vi "Parameter Set.vi"(0 "Device Type":string, 1 "Model Name":string, 3 "Interface":string(combo), 4 "Index Num":string, 5 "Parameter":string, 6 "Interface":string, 7 "Model":string) -> (2 "Data out":string[](array[string]))   [LabVIEW 2018]
panel:
  in  "Cancel":bool
  in  "OK":bool
  out "布尔 2":bool
  out "布尔":bool
  in  "Bar":bool
  in  "Address":string(combo)="1"
  in  "IP":string
  in  "IP 4":string
  in  "IP 3":string
  in  "IP 2":string
  in  "IP":string
  in  "Device Num":string(combo)="1"
  in  "Boolean":bool
  in  "Index Num":string(combo)="1"
  in  "SN":string
  in  "PID":string
  in  "VID":string
  in  "Stop Bits":string(combo)="1"
  in  "Data Bits":string(combo)="8"
  in  "Parity":u16(ring) items=["None", "Odd", "Even", "Mark", "Space"]
  in  "Baud Rate":string(combo)="9600"
  in  "COM Port":string(combo)="1"
  in  "GPIB Address":u16
  # "Drive_Parameter set"
  # "Parameter"
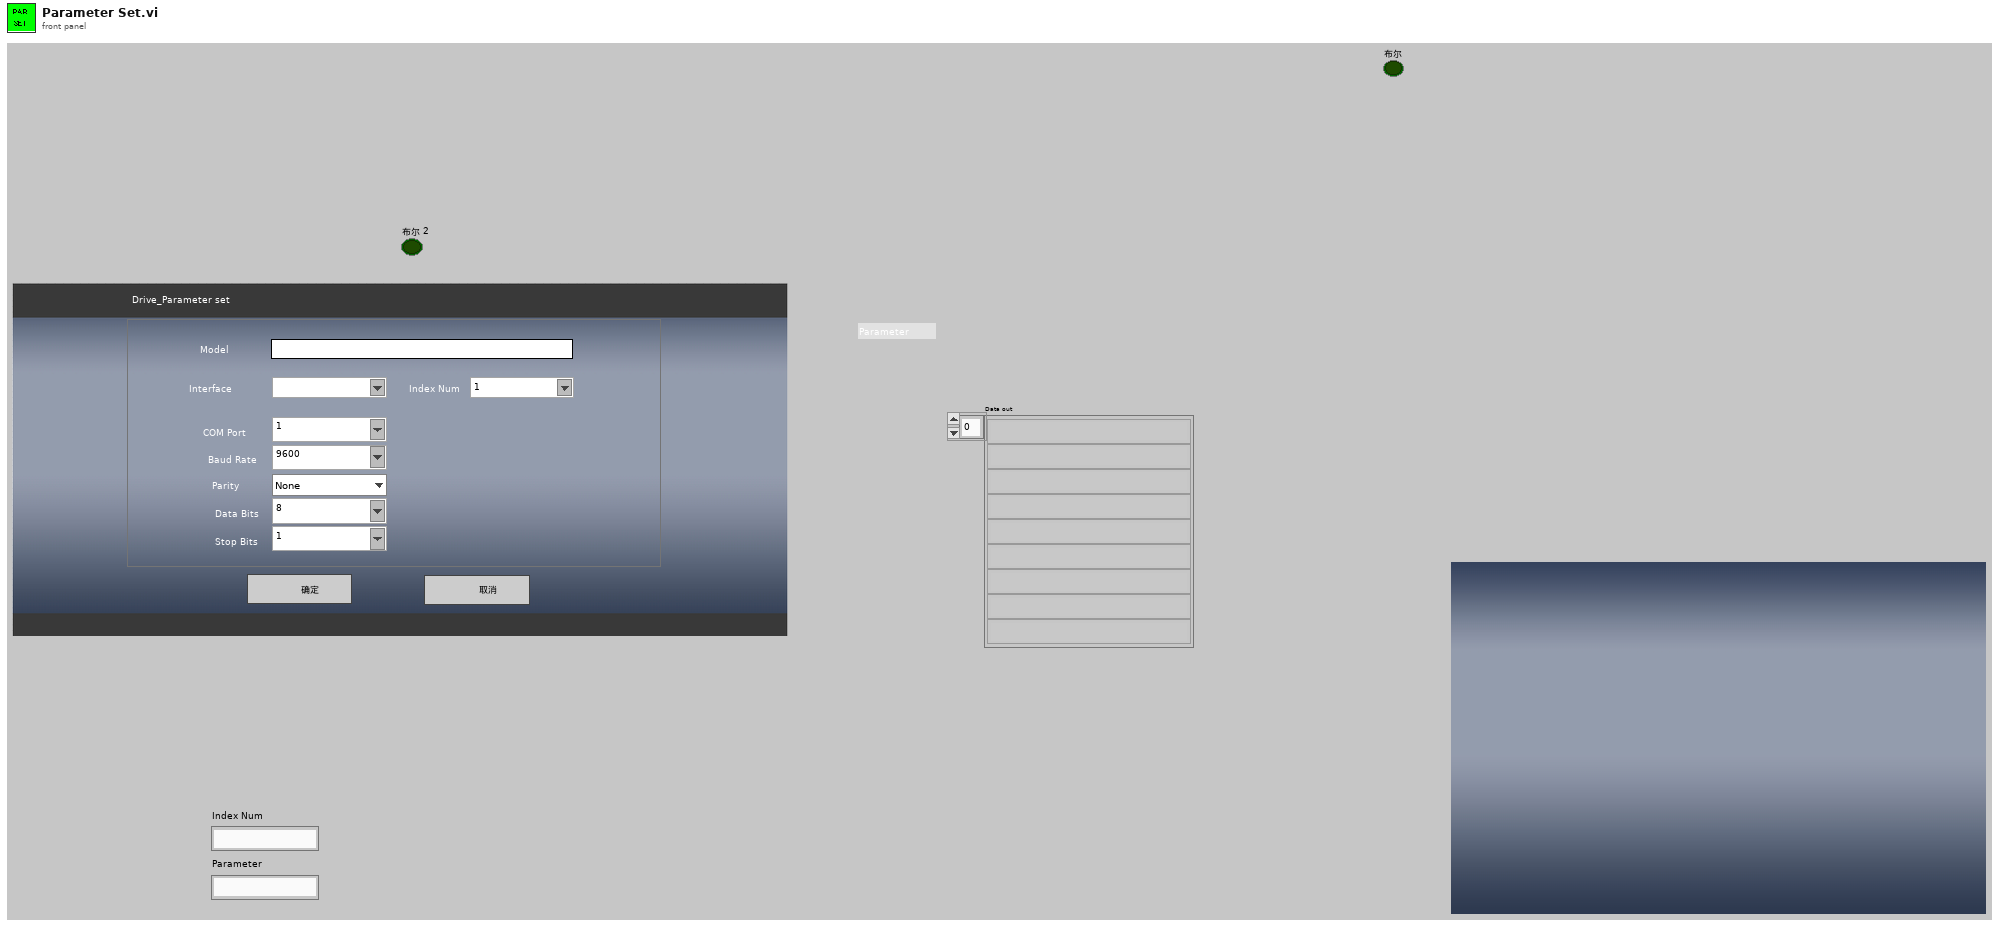
[diagram p1: front panel]
types:
  T1 = typedef "Window Refnum.ctl" = refnum<k1>
  T2 = typedef "Window Rectangle.ctl" = cluster{"left":i16, "top":i16, "right":i16, "bottom":i16}
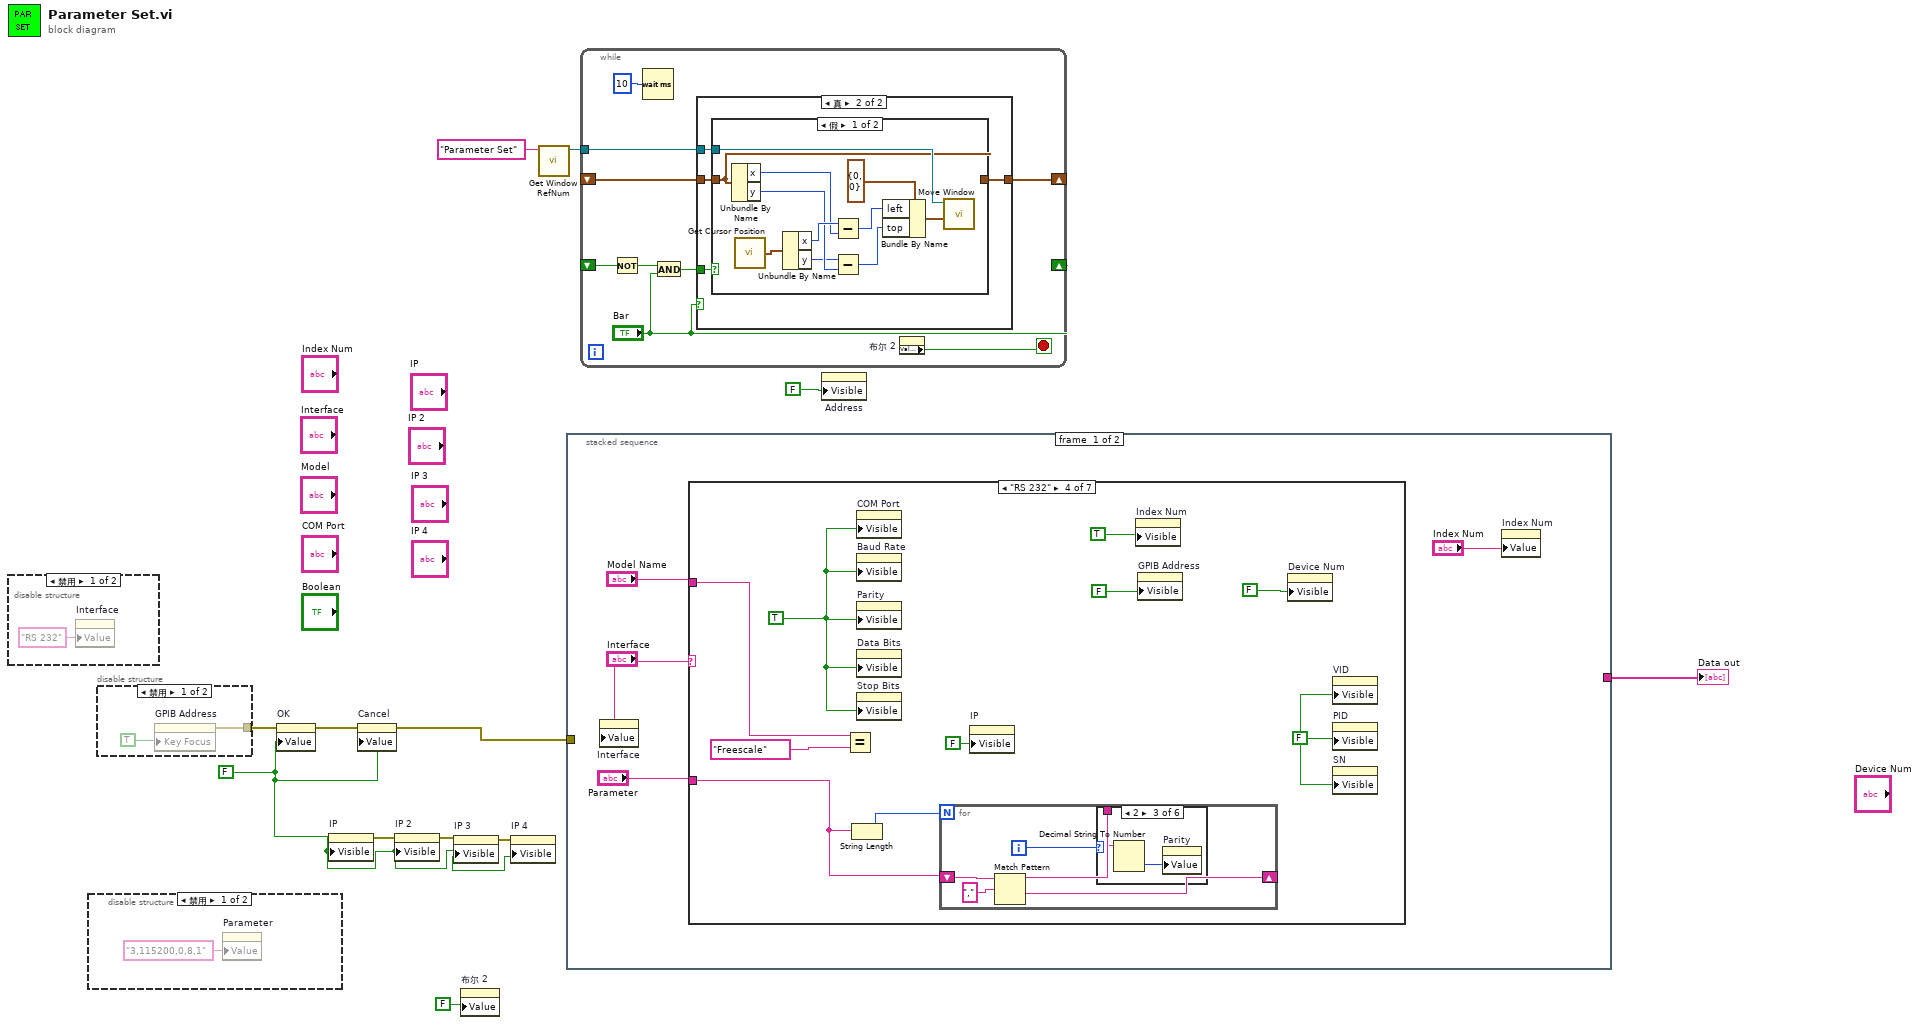
[diagram p0: block diagram]
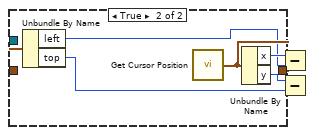
[diagram p6: hidden frame]
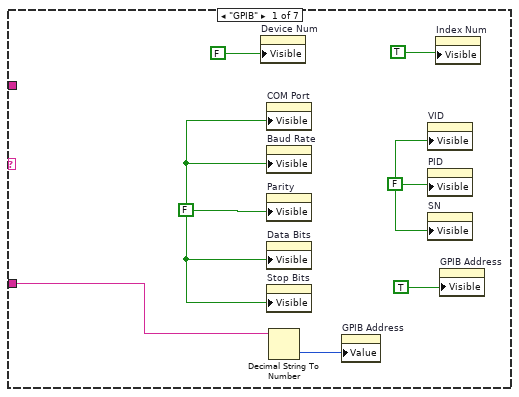
[diagram p7: hidden frame]
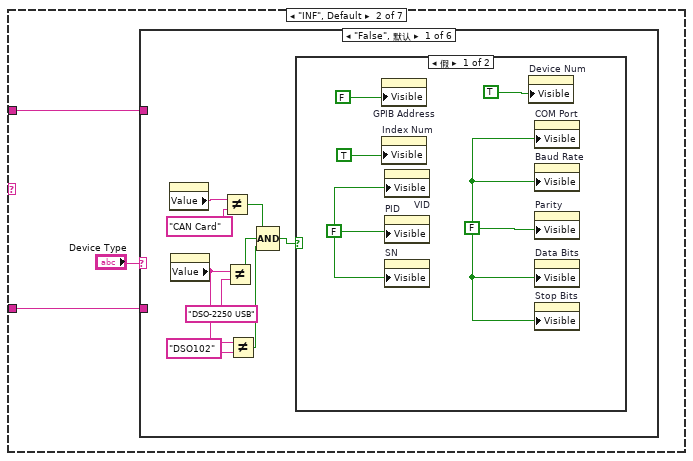
[diagram p8: hidden frame]
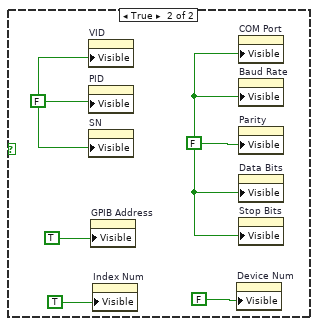
[diagram p9: hidden frame]
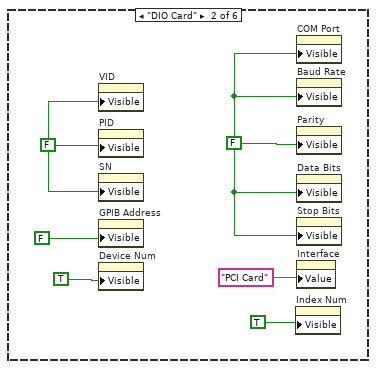
[diagram p10: hidden frame]
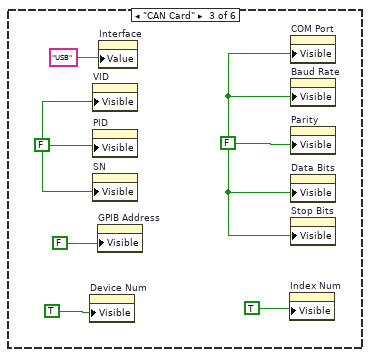
[diagram p11: hidden frame]
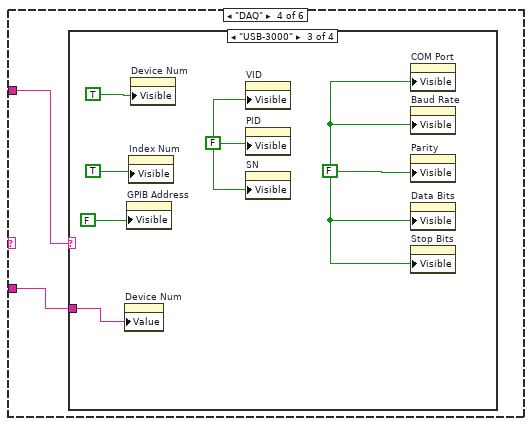
[diagram p12: hidden frame]
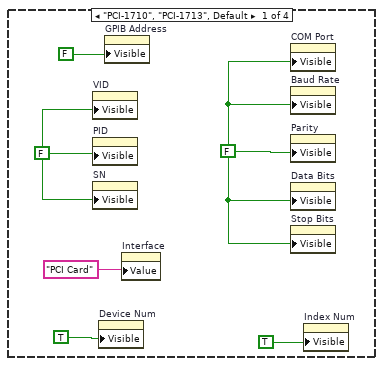
[diagram p13: hidden frame]
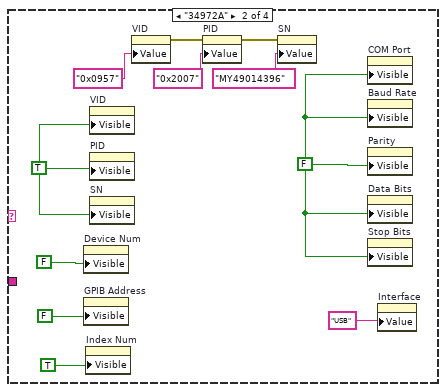
[diagram p14: hidden frame]
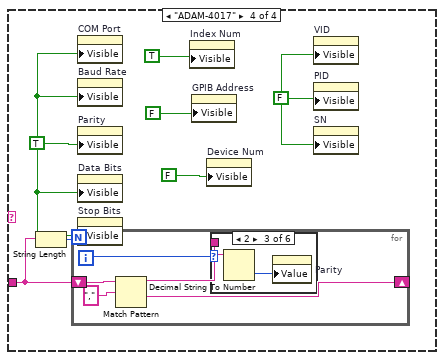
[diagram p15: hidden frame]
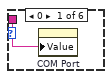
[diagram p16: hidden frame]
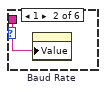
[diagram p17: hidden frame]
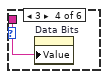
[diagram p18: hidden frame]
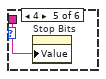
[diagram p19: hidden frame]
diagram:
  w5 = FALSE
  n1 = disable-structure shown="禁用" {
    frame Disabled {
      n2 = property on="Interface" class="Str"("Value"="RS 232" ("Interface")) -> ()  [unwired: 2 in, 2 out]
    }
    frame Enabled {
    }
  }
  n3 = disable-structure shown="禁用" {
    frame Disabled {
      n4 = property on="Parameter" class="Str"("Value"="3,115200,0,8,1" ("Parameter")) -> ()  [unwired: 2 in, 2 out]
    }
    frame Enabled {
    }
  }
  n5 = disable-structure shown="禁用" {
    disable-tunnel: [w16 _] -> w11
    frame Disabled {
      n6 = property on="GPIB Address" class="DigNum (严格)"("Key Focus"=TRUE) -> (error out=w16:errorcluster)  [unwired: 2 in, 1 out]
    }
    frame Enabled {
    }
  }
  n7 = property on="OK" class="Bool (严格)"(error in=w11, "Value"=w5) -> (error out=w12:errorcluster)  [unwired: 1 in, 1 out]
  n8 = property on="IP" class="Str"("Visible"=w5) -> (error out=w6:errorcluster)  [unwired: 2 in, 1 out]
  n9 = property on="Cancel" class="Bool (严格)"(error in=w12, "Value"=w5) -> (error out=w10:errorcluster)  [unwired: 1 in, 1 out]
  n10 = property on="IP 2" class="Str"(error in=w6, "Visible"=w5) -> (error out=w7:errorcluster)  [unwired: 1 in, 1 out]
  n11 = property on="IP 3" class="Str"(error in=w7, "Visible"=w5) -> (error out=w8:errorcluster)  [unwired: 1 in, 1 out]
  n12 = property on="布尔 2" class="Bool (严格)"("Value"=FALSE ("布尔 2")) -> ()  [unwired: 2 in, 2 out]
  n13 = property on="IP 4" class="Str"(error in=w8, "Visible"=w5) -> ()  [unwired: 1 in, 2 out]
  n14 = call "Get Window RefNum.vi"("window name (\"\")"="Parameter Set" ("window name (\"\")")) -> ("window refnum (NaWR)"=w2:T1)  [unwired: 1 in, 7 out]
  n15 = stacked-sequence {
    tunnel: w10 -> [_ w226]
    tunnel: [_ w225] -> w9
    frame #0 {
      n16 = property on="Interface" class="CmbBox"("Value"="Interface") -> ()  [unwired: 2 in, 2 out]
      n17 = case shown="\"RS 232\"" "Interface" {
        tunnel: "Parameter" -> [w23 w28 _ w149 w171 w198 w224]
        tunnel: "Model Name" -> [_ w29 _ w146 w168 w187 _]
        frame "GPIB" {
          w27 = FALSE
          w25 = FALSE
          n18 = property on="Device Num" class="CmbBox"("Visible"=FALSE) -> ()  [unwired: 2 in, 2 out]
          n19 = property on="COM Port" class="CmbBox"("Visible"=w25) -> ()  [unwired: 2 in, 2 out]
          n20 = property on="Baud Rate" class="CmbBox"("Visible"=w25) -> ()  [unwired: 2 in, 2 out]
          n21 = property on="Parity" class="Ring (严格)"("Visible"=w25) -> ()  [unwired: 2 in, 2 out]
          n22 = property on="Data Bits" class="CmbBox"("Visible"=w25) -> ()  [unwired: 2 in, 2 out]
          n23 = property on="Stop Bits" class="CmbBox"("Visible"=w25) -> ()  [unwired: 2 in, 2 out]
          n24 = Decimal String To Number(string=w23) -> (number=w24:i32)  [unwired: 3 out]
          n25 = property on="GPIB Address" class="DigNum (严格)"("Value"=w24) -> ()  [unwired: 2 in, 2 out]
          n26 = property on="VID" class="Str"("Visible"=w27) -> ()  [unwired: 2 in, 2 out]
          n27 = property on="PID" class="Str"("Visible"=w27) -> ()  [unwired: 2 in, 2 out]
          n28 = property on="SN" class="Str"("Visible"=w27) -> ()  [unwired: 2 in, 2 out]
          n29 = property on="Index Num" class="CmbBox"("Visible"=TRUE) -> ()  [unwired: 2 in, 2 out]
          n30 = property on="GPIB Address" class="DigNum (严格)"("Visible"=TRUE) -> ()  [unwired: 2 in, 2 out]
        }
        frame "INF", Default {
          n31 = case shown="\"False\", 默认" "Device Type" {
            tunnel: w29 -> [_ _ _ w63 w105 w117]
            tunnel: w28 -> [_ _ _ w62 _ _]
            frame "False", Default {
              n32 = property on="Device Type" class="Str"() -> ("Value"=w37:string)  [unwired: 2 in, 2 out]
              n33 = property on="Model Name" class="Str"() -> ("Value"=w34:string)  [unwired: 2 in, 2 out]
              n34 = Not Equal?(x=w37, y="CAN Card") -> (x != y?=w36:bool)
              n35 = Not Equal?(x=w34, y="DSO-2250 USB") -> (x != y?=w35:bool)
              n36 = Not Equal?(x=w34, y="DSO102") -> (x != y?=w32:bool)
              n37 = Compound Arithmetic op=AND(w36, w35, w32) -> (w31:bool)
              n38 = case shown="假" w31 {
                frame False {
                  w43 = FALSE
                  w44 = FALSE
                  n39 = property on="GPIB Address" class="DigNum (严格)"("Visible"=FALSE) -> ()  [unwired: 2 in, 2 out]
                  n40 = property on="Index Num" class="CmbBox"("Visible"=TRUE) -> ()  [unwired: 2 in, 2 out]
                  n41 = property on="VID" class="Str"("Visible"=w44) -> ()  [unwired: 2 in, 2 out]
                  n42 = property on="PID" class="Str"("Visible"=w44) -> ()  [unwired: 2 in, 2 out]
                  n43 = property on="SN" class="Str"("Visible"=w44) -> ()  [unwired: 2 in, 2 out]
                  n44 = property on="Device Num" class="CmbBox"("Visible"=TRUE) -> ()  [unwired: 2 in, 2 out]
                  n45 = property on="COM Port" class="CmbBox"("Visible"=w43) -> ()  [unwired: 2 in, 2 out]
                  n46 = property on="Baud Rate" class="CmbBox"("Visible"=w43) -> ()  [unwired: 2 in, 2 out]
                  n47 = property on="Parity" class="Ring (严格)"("Visible"=w43) -> ()  [unwired: 2 in, 2 out]
                  n48 = property on="Data Bits" class="CmbBox"("Visible"=w43) -> ()  [unwired: 2 in, 2 out]
                  n49 = property on="Stop Bits" class="CmbBox"("Visible"=w43) -> ()  [unwired: 2 in, 2 out]
                }
                frame True {
                  w48 = FALSE
                  w49 = FALSE
                  n50 = property on="VID" class="Str"("Visible"=w49) -> ()  [unwired: 2 in, 2 out]
                  n51 = property on="PID" class="Str"("Visible"=w49) -> ()  [unwired: 2 in, 2 out]
                  n52 = property on="SN" class="Str"("Visible"=w49) -> ()  [unwired: 2 in, 2 out]
                  n53 = property on="GPIB Address" class="DigNum (严格)"("Visible"=TRUE) -> ()  [unwired: 2 in, 2 out]
                  n54 = property on="Index Num" class="CmbBox"("Visible"=TRUE) -> ()  [unwired: 2 in, 2 out]
                  n55 = property on="Device Num" class="CmbBox"("Visible"=FALSE) -> ()  [unwired: 2 in, 2 out]
                  n56 = property on="COM Port" class="CmbBox"("Visible"=w48) -> ()  [unwired: 2 in, 2 out]
                  n57 = property on="Baud Rate" class="CmbBox"("Visible"=w48) -> ()  [unwired: 2 in, 2 out]
                  n58 = property on="Parity" class="Ring (严格)"("Visible"=w48) -> ()  [unwired: 2 in, 2 out]
                  n59 = property on="Data Bits" class="CmbBox"("Visible"=w48) -> ()  [unwired: 2 in, 2 out]
                  n60 = property on="Stop Bits" class="CmbBox"("Visible"=w48) -> ()  [unwired: 2 in, 2 out]
                }
              }
            }
            frame "DIO Card" {
              w54 = FALSE
              w55 = FALSE
              n61 = property on="VID" class="Str"("Visible"=w55) -> ()  [unwired: 2 in, 2 out]
              n62 = property on="PID" class="Str"("Visible"=w55) -> ()  [unwired: 2 in, 2 out]
              n63 = property on="SN" class="Str"("Visible"=w55) -> ()  [unwired: 2 in, 2 out]
              n64 = property on="GPIB Address" class="DigNum (严格)"("Visible"=FALSE) -> ()  [unwired: 2 in, 2 out]
              n65 = property on="Device Num" class="CmbBox"("Visible"=TRUE) -> ()  [unwired: 2 in, 2 out]
              n66 = property on="Index Num" class="CmbBox"("Visible"=TRUE) -> ()  [unwired: 2 in, 2 out]
              n67 = property on="COM Port" class="CmbBox"("Visible"=w54) -> ()  [unwired: 2 in, 2 out]
              n68 = property on="Baud Rate" class="CmbBox"("Visible"=w54) -> ()  [unwired: 2 in, 2 out]
              n69 = property on="Parity" class="Ring (严格)"("Visible"=w54) -> ()  [unwired: 2 in, 2 out]
              n70 = property on="Data Bits" class="CmbBox"("Visible"=w54) -> ()  [unwired: 2 in, 2 out]
              n71 = property on="Stop Bits" class="CmbBox"("Visible"=w54) -> ()  [unwired: 2 in, 2 out]
              n72 = property on="Interface" class="CmbBox"("Value"="PCI Card" ("Interface")) -> ()  [unwired: 2 in, 2 out]
            }
            frame "CAN Card" {
              w60 = FALSE
              w61 = FALSE
              n73 = property on="Device Num" class="CmbBox"("Visible"=TRUE) -> ()  [unwired: 2 in, 2 out]
              n74 = property on="VID" class="Str"("Visible"=w61) -> ()  [unwired: 2 in, 2 out]
              n75 = property on="PID" class="Str"("Visible"=w61) -> ()  [unwired: 2 in, 2 out]
              n76 = property on="SN" class="Str"("Visible"=w61) -> ()  [unwired: 2 in, 2 out]
              n77 = property on="GPIB Address" class="DigNum (严格)"("Visible"=FALSE) -> ()  [unwired: 2 in, 2 out]
              n78 = property on="Interface" class="CmbBox"("Value"="USB" ("Interface")) -> ()  [unwired: 2 in, 2 out]
              n79 = property on="Index Num" class="CmbBox"("Visible"=TRUE) -> ()  [unwired: 2 in, 2 out]
              n80 = property on="COM Port" class="CmbBox"("Visible"=w60) -> ()  [unwired: 2 in, 2 out]
              n81 = property on="Baud Rate" class="CmbBox"("Visible"=w60) -> ()  [unwired: 2 in, 2 out]
              n82 = property on="Parity" class="Ring (严格)"("Visible"=w60) -> ()  [unwired: 2 in, 2 out]
              n83 = property on="Data Bits" class="CmbBox"("Visible"=w60) -> ()  [unwired: 2 in, 2 out]
              n84 = property on="Stop Bits" class="CmbBox"("Visible"=w60) -> ()  [unwired: 2 in, 2 out]
            }
            frame "DAQ" {
              n85 = case shown="\"USB-3000\"" w63 {
                tunnel: w62 -> [_ _ w81 w87]
                frame "PCI-1710", "PCI-1713", Default {
                  w68 = FALSE
                  w69 = FALSE
                  n86 = property on="VID" class="Str"("Visible"=w69) -> ()  [unwired: 2 in, 2 out]
                  n87 = property on="PID" class="Str"("Visible"=w69) -> ()  [unwired: 2 in, 2 out]
                  n88 = property on="SN" class="Str"("Visible"=w69) -> ()  [unwired: 2 in, 2 out]
                  n89 = property on="Device Num" class="CmbBox"("Visible"=TRUE) -> ()  [unwired: 2 in, 2 out]
                  n90 = property on="GPIB Address" class="DigNum (严格)"("Visible"=FALSE) -> ()  [unwired: 2 in, 2 out]
                  n91 = property on="Interface" class="CmbBox"("Value"="PCI Card" ("Interface")) -> ()  [unwired: 2 in, 2 out]
                  n92 = property on="COM Port" class="CmbBox"("Visible"=w68) -> ()  [unwired: 2 in, 2 out]
                  n93 = property on="Baud Rate" class="CmbBox"("Visible"=w68) -> ()  [unwired: 2 in, 2 out]
                  n94 = property on="Parity" class="Ring (严格)"("Visible"=w68) -> ()  [unwired: 2 in, 2 out]
                  n95 = property on="Data Bits" class="CmbBox"("Visible"=w68) -> ()  [unwired: 2 in, 2 out]
                  n96 = property on="Stop Bits" class="CmbBox"("Visible"=w68) -> ()  [unwired: 2 in, 2 out]
                  n97 = property on="Index Num" class="CmbBox"("Visible"=TRUE) -> ()  [unwired: 2 in, 2 out]
                }
                frame "34972A" {
                  w79 = FALSE
                  w80 = TRUE
                  n98 = property on="Device Num" class="CmbBox"("Visible"=FALSE) -> ()  [unwired: 2 in, 2 out]
                  n99 = property on="GPIB Address" class="DigNum (严格)"("Visible"=FALSE) -> ()  [unwired: 2 in, 2 out]
                  n100 = property on="Index Num" class="CmbBox"("Visible"=TRUE) -> ()  [unwired: 2 in, 2 out]
                  n101 = property on="VID" class="Str"("Visible"=w80) -> ()  [unwired: 2 in, 2 out]
                  n102 = property on="PID" class="Str"("Visible"=w80) -> ()  [unwired: 2 in, 2 out]
                  n103 = property on="SN" class="Str"("Visible"=w80) -> ()  [unwired: 2 in, 2 out]
                  n104 = property on="VID" class="Str"("Value"="0x0957" ("VID")) -> (error out=w75:errorcluster)  [unwired: 2 in, 1 out]
                  n105 = property on="PID" class="Str"(error in=w75, "Value"="0x2007" ("PID")) -> (error out=w73:errorcluster)  [unwired: 1 in, 1 out]
                  n106 = property on="SN" class="Str"(error in=w73, "Value"="MY49014396" ("SN")) -> ()  [unwired: 1 in, 2 out]
                  n107 = property on="COM Port" class="CmbBox"("Visible"=w79) -> ()  [unwired: 2 in, 2 out]
                  n108 = property on="Baud Rate" class="CmbBox"("Visible"=w79) -> ()  [unwired: 2 in, 2 out]
                  n109 = property on="Parity" class="Ring (严格)"("Visible"=w79) -> ()  [unwired: 2 in, 2 out]
                  n110 = property on="Data Bits" class="CmbBox"("Visible"=w79) -> ()  [unwired: 2 in, 2 out]
                  n111 = property on="Stop Bits" class="CmbBox"("Visible"=w79) -> ()  [unwired: 2 in, 2 out]
                  n112 = property on="Interface" class="CmbBox"("Value"="USB" ("Interface")) -> ()  [unwired: 2 in, 2 out]
                }
                frame "USB-3000" {
                  w83 = FALSE
                  w84 = FALSE
                  n113 = property on="Device Num" class="CmbBox"("Value"=w81) -> ()  [unwired: 2 in, 2 out]
                  n114 = property on="GPIB Address" class="DigNum (严格)"("Visible"=FALSE) -> ()  [unwired: 2 in, 2 out]
                  n115 = property on="Index Num" class="CmbBox"("Visible"=TRUE) -> ()  [unwired: 2 in, 2 out]
                  n116 = property on="Device Num" class="CmbBox"("Visible"=TRUE) -> ()  [unwired: 2 in, 2 out]
                  n117 = property on="VID" class="Str"("Visible"=w83) -> ()  [unwired: 2 in, 2 out]
                  n118 = property on="PID" class="Str"("Visible"=w83) -> ()  [unwired: 2 in, 2 out]
                  n119 = property on="SN" class="Str"("Visible"=w83) -> ()  [unwired: 2 in, 2 out]
                  n120 = property on="COM Port" class="CmbBox"("Visible"=w84) -> ()  [unwired: 2 in, 2 out]
                  n121 = property on="Baud Rate" class="CmbBox"("Visible"=w84) -> ()  [unwired: 2 in, 2 out]
                  n122 = property on="Parity" class="Ring (严格)"("Visible"=w84) -> ()  [unwired: 2 in, 2 out]
                  n123 = property on="Data Bits" class="CmbBox"("Visible"=w84) -> ()  [unwired: 2 in, 2 out]
                  n124 = property on="Stop Bits" class="CmbBox"("Visible"=w84) -> ()  [unwired: 2 in, 2 out]
                }
                frame "ADAM-4017" {
                  w91 = FALSE
                  w93 = TRUE
                  n125 = String Length(string=w87) -> (length=w88:i32)
                  n126 = for {
                    N: w88 -> [_]
                    shift-right: [w96] -> _
                    shift-left: w87 -> [w98]
                    i -> [w95]
                    n127 = Match Pattern(string=w98, regular expression=",") -> (before substring=w94:string, after substring=w96:string)  [unwired: 3 out]
                    n128 = case shown="2" w95 {
                      tunnel: w94 -> [w99 w100 w102 w103 w104 _]
                      frame 0 {
                        n129 = property on="COM Port" class="CmbBox"("Value"=w99) -> ()  [unwired: 2 in, 2 out]
                      }
                      frame 1 {
                        n130 = property on="Baud Rate" class="CmbBox"("Value"=w100) -> ()  [unwired: 2 in, 2 out]
                      }
                      frame 2 {
                        n131 = Decimal String To Number(string=w102) -> (number=w101:i32)  [unwired: 3 out]
                        n132 = property on="Parity" class="Ring (严格)"("Value"=w101) -> ()  [unwired: 2 in, 2 out]
                      }
                      frame 3 {
                        n133 = property on="Data Bits" class="CmbBox"("Value"=w103) -> ()  [unwired: 2 in, 2 out]
                      }
                      frame 4 {
                        n134 = property on="Stop Bits" class="CmbBox"("Value"=w104) -> ()  [unwired: 2 in, 2 out]
                      }
                      frame 5, Default {
                      }
                    }
                  }
                  n135 = property on="COM Port" class="CmbBox"("Visible"=w93) -> ()  [unwired: 2 in, 2 out]
                  n136 = property on="Baud Rate" class="CmbBox"("Visible"=w93) -> ()  [unwired: 2 in, 2 out]
                  n137 = property on="Parity" class="Ring (严格)"("Visible"=w93) -> ()  [unwired: 2 in, 2 out]
                  n138 = property on="Data Bits" class="CmbBox"("Visible"=w93) -> ()  [unwired: 2 in, 2 out]
                  n139 = property on="Stop Bits" class="CmbBox"("Visible"=w93) -> ()  [unwired: 2 in, 2 out]
                  n140 = property on="Index Num" class="CmbBox"("Visible"=TRUE) -> ()  [unwired: 2 in, 2 out]
                  n141 = property on="GPIB Address" class="DigNum (严格)"("Visible"=FALSE) -> ()  [unwired: 2 in, 2 out]
                  n142 = property on="Device Num" class="CmbBox"("Visible"=FALSE) -> ()  [unwired: 2 in, 2 out]
                  n143 = property on="VID" class="Str"("Visible"=w91) -> ()  [unwired: 2 in, 2 out]
                  n144 = property on="PID" class="Str"("Visible"=w91) -> ()  [unwired: 2 in, 2 out]
                  n145 = property on="SN" class="Str"("Visible"=w91) -> ()  [unwired: 2 in, 2 out]
                }
              }
            }
            frame "Power Aanalysis Meter" {
              n146 = case shown="\"66202\"" w105 {
                frame "66202" {
                  w115 = FALSE
                  w116 = TRUE
                  n147 = property on="VID" class="Str"("Visible"=w116) -> ()  [unwired: 2 in, 2 out]
                  n148 = property on="PID" class="Str"("Visible"=w116) -> ()  [unwired: 2 in, 2 out]
                  n149 = property on="SN" class="Str"("Visible"=w116) -> ()  [unwired: 2 in, 2 out]
                  n150 = property on="VID" class="Str"("Value"="0x0A69" ("VID")) -> (error out=w111:errorcluster)  [unwired: 2 in, 1 out]
                  n151 = property on="PID" class="Str"(error in=w111, "Value"="0x0835" ("PID")) -> (error out=w109:errorcluster)  [unwired: 1 in, 1 out]
                  n152 = property on="Device Num" class="CmbBox"("Visible"=FALSE) -> ()  [unwired: 2 in, 2 out]
                  n153 = property on="GPIB Address" class="DigNum (严格)"("Visible"=FALSE) -> ()  [unwired: 2 in, 2 out]
                  n154 = property on="Index Num" class="CmbBox"("Visible"=TRUE) -> ()  [unwired: 2 in, 2 out]
                  n155 = property on="SN" class="Str"(error in=w109, "Value"="A66200110136" ("SN")) -> ()  [unwired: 1 in, 2 out]
                  n156 = property on="COM Port" class="CmbBox"("Visible"=w115) -> ()  [unwired: 2 in, 2 out]
                  n157 = property on="Baud Rate" class="CmbBox"("Visible"=w115) -> ()  [unwired: 2 in, 2 out]
                  n158 = property on="Parity" class="Ring (严格)"("Visible"=w115) -> ()  [unwired: 2 in, 2 out]
                  n159 = property on="Data Bits" class="CmbBox"("Visible"=w115) -> ()  [unwired: 2 in, 2 out]
                  n160 = property on="Stop Bits" class="CmbBox"("Visible"=w115) -> ()  [unwired: 2 in, 2 out]
                  n161 = property on="Interface" class="CmbBox"("Value"="USB" ("Interface")) -> ()  [unwired: 2 in, 2 out]
                }
                frame "false", Default {
                }
              }
            }
            frame "Oscilloscope" {
              n162 = case shown="\"DPO-3054\"" w117 {
                frame "DPO-3054" {
                  w127 = FALSE
                  w128 = TRUE
                  n163 = property on="Device Num" class="CmbBox"("Visible"=FALSE) -> ()  [unwired: 2 in, 2 out]
                  n164 = property on="VID" class="Str"("Visible"=w128) -> ()  [unwired: 2 in, 2 out]
                  n165 = property on="PID" class="Str"("Visible"=w128) -> ()  [unwired: 2 in, 2 out]
                  n166 = property on="SN" class="Str"("Visible"=w128) -> ()  [unwired: 2 in, 2 out]
                  n167 = property on="VID" class="Str"("Value"="0x0699" ("VID")) -> (error out=w123:errorcluster)  [unwired: 2 in, 1 out]
                  n168 = property on="PID" class="Str"(error in=w123, "Value"="0x0415" ("PID")) -> (error out=w121:errorcluster)  [unwired: 1 in, 1 out]
                  n169 = property on="GPIB Address" class="DigNum (严格)"("Visible"=FALSE) -> ()  [unwired: 2 in, 2 out]
                  n170 = property on="Index Num" class="CmbBox"("Visible"=TRUE) -> ()  [unwired: 2 in, 2 out]
                  n171 = property on="SN" class="Str"(error in=w121, "Value"="C030431" ("SN")) -> ()  [unwired: 1 in, 2 out]
                  n172 = property on="COM Port" class="CmbBox"("Visible"=w127) -> ()  [unwired: 2 in, 2 out]
                  n173 = property on="Baud Rate" class="CmbBox"("Visible"=w127) -> ()  [unwired: 2 in, 2 out]
                  n174 = property on="Parity" class="Ring (严格)"("Visible"=w127) -> ()  [unwired: 2 in, 2 out]
                  n175 = property on="Data Bits" class="CmbBox"("Visible"=w127) -> ()  [unwired: 2 in, 2 out]
                  n176 = property on="Stop Bits" class="CmbBox"("Visible"=w127) -> ()  [unwired: 2 in, 2 out]
                  n177 = property on="Interface" class="CmbBox"("Value"="USB" ("Interface")) -> ()  [unwired: 2 in, 2 out]
                }
                frame "TDS 2014C" {
                  w138 = FALSE
                  w139 = TRUE
                  n178 = property on="Interface" class="CmbBox"("Value"="USB" ("Interface")) -> ()  [unwired: 2 in, 2 out]
                  n179 = property on="VID" class="Str"("Visible"=w139) -> ()  [unwired: 2 in, 2 out]
                  n180 = property on="PID" class="Str"("Visible"=w139) -> ()  [unwired: 2 in, 2 out]
                  n181 = property on="SN" class="Str"("Visible"=w139) -> ()  [unwired: 2 in, 2 out]
                  n182 = property on="VID" class="Str"("Value"="0x0699" ("VID")) -> (error out=w134:errorcluster)  [unwired: 2 in, 1 out]
                  n183 = property on="PID" class="Str"(error in=w134, "Value"="0x03A4" ("PID")) -> (error out=w132:errorcluster)  [unwired: 1 in, 1 out]
                  n184 = property on="Device Num" class="CmbBox"("Visible"=FALSE) -> ()  [unwired: 2 in, 2 out]
                  n185 = property on="GPIB Address" class="DigNum (严格)"("Visible"=FALSE) -> ()  [unwired: 2 in, 2 out]
                  n186 = property on="Index Num" class="CmbBox"("Visible"=TRUE) -> ()  [unwired: 2 in, 2 out]
                  n187 = property on="SN" class="Str"(error in=w132, "Value"="C030830" ("SN")) -> ()  [unwired: 1 in, 2 out]
                  n188 = property on="COM Port" class="CmbBox"("Visible"=w138) -> ()  [unwired: 2 in, 2 out]
                  n189 = property on="Baud Rate" class="CmbBox"("Visible"=w138) -> ()  [unwired: 2 in, 2 out]
                  n190 = property on="Parity" class="Ring (严格)"("Visible"=w138) -> ()  [unwired: 2 in, 2 out]
                  n191 = property on="Data Bits" class="CmbBox"("Visible"=w138) -> ()  [unwired: 2 in, 2 out]
                  n192 = property on="Stop Bits" class="CmbBox"("Visible"=w138) -> ()  [unwired: 2 in, 2 out]
                }
                frame "false", Default {
                }
              }
            }
          }
        }
        frame "TCP" {
          w140 = TRUE
          # "读取程式中设定的值到选择框"
          n193 = property on="IP" class="Str"("Visible"=w140) -> (error out=w143:errorcluster)  [unwired: 2 in, 1 out]
          n194 = property on="IP 2" class="Str"(error in=w143, "Visible"=w140) -> (error out=w142:errorcluster)  [unwired: 1 in, 1 out]
          n195 = property on="IP 3" class="Str"(error in=w142, "Visible"=w140) -> (error out=w141:errorcluster)  [unwired: 1 in, 1 out]
          n196 = property on="IP 4" class="Str"(error in=w141, "Visible"=w140) -> ()  [unwired: 1 in, 2 out]
        }
        frame "RS 232" {
          w151 = FALSE
          w153 = TRUE
          n197 = Equal?(x=w146, y="Freescale") -> ()  [unwired: 1 out]
          n198 = String Length(string=w149) -> (length=w150:i32)
          n199 = property on="COM Port" class="CmbBox"("Visible"=w153) -> ()  [unwired: 2 in, 2 out]
          n200 = property on="Baud Rate" class="CmbBox"("Visible"=w153) -> ()  [unwired: 2 in, 2 out]
          n201 = property on="Parity" class="Ring (严格)"("Visible"=w153) -> ()  [unwired: 2 in, 2 out]
          n202 = property on="Data Bits" class="CmbBox"("Visible"=w153) -> ()  [unwired: 2 in, 2 out]
          n203 = property on="Stop Bits" class="CmbBox"("Visible"=w153) -> ()  [unwired: 2 in, 2 out]
          n204 = for {
            N: w150 -> [_]
            shift-right: [w156] -> _
            shift-left: w149 -> [w158]
            i -> [w155]
            n205 = Match Pattern(string=w158, regular expression=",") -> (before substring=w154:string, after substring=w156:string)  [unwired: 3 out]
            n206 = case shown="2" w155 {
              tunnel: w154 -> [w159 w160 w162 w163 w164 _]
              frame 0 {
                n207 = property on="COM Port" class="CmbBox"("Value"=w159) -> ()  [unwired: 2 in, 2 out]
              }
              frame 1 {
                n208 = property on="Baud Rate" class="CmbBox"("Value"=w160) -> ()  [unwired: 2 in, 2 out]
              }
              frame 2 {
                n209 = Decimal String To Number(string=w162) -> (number=w161:i32)  [unwired: 3 out]
                n210 = property on="Parity" class="Ring (严格)"("Value"=w161) -> ()  [unwired: 2 in, 2 out]
              }
              frame 3 {
                n211 = property on="Data Bits" class="CmbBox"("Value"=w163) -> ()  [unwired: 2 in, 2 out]
              }
              frame 4 {
                n212 = property on="Stop Bits" class="CmbBox"("Value"=w164) -> ()  [unwired: 2 in, 2 out]
              }
              frame 5, Default {
              }
            }
          }
          n213 = property on="IP" class="Str"("Visible"=FALSE ("可见")) -> ()  [unwired: 2 in, 2 out]
          n214 = property on="Index Num" class="CmbBox"("Visible"=TRUE) -> ()  [unwired: 2 in, 2 out]
          n215 = property on="GPIB Address" class="DigNum (严格)"("Visible"=FALSE) -> ()  [unwired: 2 in, 2 out]
          n216 = property on="Device Num" class="CmbBox"("Visible"=FALSE) -> ()  [unwired: 2 in, 2 out]
          n217 = property on="VID" class="Str"("Visible"=w151) -> ()  [unwired: 2 in, 2 out]
          n218 = property on="PID" class="Str"("Visible"=w151) -> ()  [unwired: 2 in, 2 out]
          n219 = property on="SN" class="Str"("Visible"=w151) -> ()  [unwired: 2 in, 2 out]
        }
        frame "RS 485" {
          w173 = FALSE
          w165 = TRUE
          n220 = String Length(string=w171) -> (length=w172:i32)
          n221 = Equal?(x=w168, y="Freescale") -> (x = y?=w166:bool)
          n222 = property on="COM Port" class="CmbBox"("Visible"=w165) -> ()  [unwired: 2 in, 2 out]
          n223 = property on="Baud Rate" class="CmbBox"("Visible"=w165) -> ()  [unwired: 2 in, 2 out]
          n224 = property on="Parity" class="Ring (严格)"("Visible"=w165) -> ()  [unwired: 2 in, 2 out]
          n225 = property on="Data Bits" class="CmbBox"("Visible"=w165) -> ()  [unwired: 2 in, 2 out]
          n226 = property on="Stop Bits" class="CmbBox"("Visible"=w165) -> ()  [unwired: 2 in, 2 out]
          n227 = for {
            N: w172 -> [_]
            shift-right: [w177] -> _
            shift-left: w171 -> [w179]
            i -> [w176]
            n228 = Match Pattern(string=w179, regular expression=",") -> (before substring=w175:string, after substring=w177:string)  [unwired: 3 out]
            n229 = case shown="0" w176 {
              tunnel: w175 -> [w180 w181 w183 w184 w185 _]
              frame 0 {
                n230 = property on="COM Port" class="CmbBox"("Value"=w180) -> ()  [unwired: 2 in, 2 out]
              }
              frame 1 {
                n231 = property on="Baud Rate" class="CmbBox"("Value"=w181) -> ()  [unwired: 2 in, 2 out]
              }
              frame 2 {
                n232 = Decimal String To Number(string=w183) -> (number=w182:i32)  [unwired: 3 out]
                n233 = property on="Parity" class="Ring (严格)"("Value"=w182) -> ()  [unwired: 2 in, 2 out]
              }
              frame 3 {
                n234 = property on="Data Bits" class="CmbBox"("Value"=w184) -> ()  [unwired: 2 in, 2 out]
              }
              frame 4 {
                n235 = property on="Stop Bits" class="CmbBox"("Value"=w185) -> ()  [unwired: 2 in, 2 out]
              }
              frame 5, Default {
              }
            }
          }
          n236 = property on="Address" class="CmbBox"("Visible"=w165) -> ()  [unwired: 2 in, 2 out]
          n237 = property on="IP" class="Str"("Visible"=w166) -> ()  [unwired: 2 in, 2 out]
          n238 = property on="Index Num" class="CmbBox"("Visible"=TRUE) -> ()  [unwired: 2 in, 2 out]
          n239 = property on="GPIB Address" class="DigNum (严格)"("Visible"=FALSE) -> ()  [unwired: 2 in, 2 out]
          n240 = property on="Device Num" class="CmbBox"("Visible"=FALSE) -> ()  [unwired: 2 in, 2 out]
          n241 = property on="VID" class="Str"("Visible"=w173) -> ()  [unwired: 2 in, 2 out]
          n242 = property on="PID" class="Str"("Visible"=w173) -> ()  [unwired: 2 in, 2 out]
          n243 = property on="SN" class="Str"("Visible"=w173) -> ()  [unwired: 2 in, 2 out]
        }
        frame "USB" {
          n244 = property on="Device Type" class="Str"() -> ("Value"=w195:string)  [unwired: 2 in, 2 out]
          n245 = property on="Model Name" class="Str"() -> ("Value"=w192:string)  [unwired: 2 in, 2 out]
          n246 = Equal?(x=w187, y="Freescale") -> (x = y?=w186:bool)
          n247 = Not Equal?(x=w195, y="CAN Card") -> (x != y?=w194:bool)
          n248 = Not Equal?(x=w192, y="DSO102") -> (x != y?=w190:bool)
          n249 = Not Equal?(x=w192, y="DSO-2250 USB") -> (x != y?=w193:bool)
          n250 = property on="IP" class="Str"("Visible"=w186) -> ()  [unwired: 2 in, 2 out]
          n251 = Compound Arithmetic op=AND(w194, w193, w190) -> (w189:bool)
          n252 = case shown="真" w189 {
            tunnel: w198 -> [_ w206]
            frame False {
              w201 = FALSE
              w203 = FALSE
              n253 = property on="Index Num" class="CmbBox"("Visible"=TRUE) -> ()  [unwired: 2 in, 2 out]
              n254 = property on="VID" class="Str"("Visible"=w203) -> ()  [unwired: 2 in, 2 out]
              n255 = property on="PID" class="Str"("Visible"=w203) -> ()  [unwired: 2 in, 2 out]
              n256 = property on="SN" class="Str"("Visible"=w203) -> ()  [unwired: 2 in, 2 out]
              n257 = property on="GPIB Address" class="DigNum (严格)"("Visible"=FALSE) -> ()  [unwired: 2 in, 2 out]
              n258 = property on="Device Num" class="CmbBox"("Visible"=TRUE) -> ()  [unwired: 2 in, 2 out]
              n259 = property on="COM Port" class="CmbBox"("Visible"=w201) -> ()  [unwired: 2 in, 2 out]
              n260 = property on="Baud Rate" class="CmbBox"("Visible"=w201) -> ()  [unwired: 2 in, 2 out]
              n261 = property on="Parity" class="Ring (严格)"("Visible"=w201) -> ()  [unwired: 2 in, 2 out]
              n262 = property on="Data Bits" class="CmbBox"("Visible"=w201) -> ()  [unwired: 2 in, 2 out]
              n263 = property on="Stop Bits" class="CmbBox"("Visible"=w201) -> ()  [unwired: 2 in, 2 out]
            }
            frame True {
              w208 = FALSE
              w210 = TRUE
              n264 = String Length(string=w206) -> (length=w207:i32)
              n265 = property on="VID" class="Str"("Visible"=w210) -> ()  [unwired: 2 in, 2 out]
              n266 = property on="PID" class="Str"("Visible"=w210) -> ()  [unwired: 2 in, 2 out]
              n267 = property on="SN" class="Str"("Visible"=w210) -> ()  [unwired: 2 in, 2 out]
              n268 = property on="GPIB Address" class="DigNum (严格)"("Visible"=FALSE) -> ()  [unwired: 2 in, 2 out]
              n269 = for {
                N: w207 -> [_]
                shift-right: [w213] -> _
                shift-left: w206 -> [w215]
                i -> [w212]
                n270 = Match Pattern(string=w215, regular expression=",") -> (before substring=w211:string, after substring=w213:string)  [unwired: 3 out]
                n271 = case shown="0" w212 {
                  tunnel: w211 -> [w216 w217 w218 _ _ _]
                  frame 0 {
                    n272 = property on="VID" class="Str"("Value"=w216) -> ()  [unwired: 2 in, 2 out]
                  }
                  frame 1 {
                    n273 = property on="PID" class="Str"("Value"=w217) -> ()  [unwired: 2 in, 2 out]
                  }
                  frame 2 {
                    n274 = property on="SN" class="Str"("Value"=w218) -> ()  [unwired: 2 in, 2 out]
                  }
                  frame 3 {
                  }
                  frame 4 {
                  }
                  frame 5, Default {
                  }
                }
              }
              n275 = property on="COM Port" class="CmbBox"("Visible"=w208) -> ()  [unwired: 2 in, 2 out]
              n276 = property on="Baud Rate" class="CmbBox"("Visible"=w208) -> ()  [unwired: 2 in, 2 out]
              n277 = property on="Parity" class="Ring (严格)"("Visible"=w208) -> ()  [unwired: 2 in, 2 out]
              n278 = property on="Data Bits" class="CmbBox"("Visible"=w208) -> ()  [unwired: 2 in, 2 out]
              n279 = property on="Stop Bits" class="CmbBox"("Visible"=w208) -> ()  [unwired: 2 in, 2 out]
              n280 = property on="Index Num" class="CmbBox"("Visible"=TRUE) -> ()  [unwired: 2 in, 2 out]
              n281 = property on="Device Num" class="CmbBox"("Visible"=FALSE) -> ()  [unwired: 2 in, 2 out]
            }
          }
        }
        frame "PCI Card" {
          w220 = FALSE
          w221 = FALSE
          n282 = property on="Device Num" class="CmbBox"("Value"=w224) -> ()  [unwired: 2 in, 2 out]
          n283 = property on="GPIB Address" class="DigNum (严格)"("Visible"=FALSE) -> ()  [unwired: 2 in, 2 out]
          n284 = property on="Index Num" class="CmbBox"("Visible"=TRUE) -> ()  [unwired: 2 in, 2 out]
          n285 = property on="Device Num" class="CmbBox"("Visible"=TRUE) -> ()  [unwired: 2 in, 2 out]
          n286 = property on="VID" class="Str"("Visible"=w220) -> ()  [unwired: 2 in, 2 out]
          n287 = property on="PID" class="Str"("Visible"=w220) -> ()  [unwired: 2 in, 2 out]
          n288 = property on="SN" class="Str"("Visible"=w220) -> ()  [unwired: 2 in, 2 out]
          n289 = property on="COM Port" class="CmbBox"("Visible"=w221) -> ()  [unwired: 2 in, 2 out]
          n290 = property on="Baud Rate" class="CmbBox"("Visible"=w221) -> ()  [unwired: 2 in, 2 out]
          n291 = property on="Parity" class="Ring (严格)"("Visible"=w221) -> ()  [unwired: 2 in, 2 out]
          n292 = property on="Data Bits" class="CmbBox"("Visible"=w221) -> ()  [unwired: 2 in, 2 out]
          n293 = property on="Stop Bits" class="CmbBox"("Visible"=w221) -> ()  [unwired: 2 in, 2 out]
        }
      }
      n294 = property on="Index Num" class="CmbBox"("Value"="Index Num") -> ()  [unwired: 2 in, 2 out]
    }
    frame #1 {
      n295 = while {
        tunnel: w226 -> [_]
        tunnel: [w227] -> w225
        stop <- w228 stop-if-true
        n296 = event shown="[1] \"Interface\": 值改变" {
          selector: _ -> [_ _ _]
          dyn-events: _ -> [_ _ _]
          timeout: _ -> [_ _ _]
          tunnel: [TRUE _ TRUE] -> w228
          tunnel: [w233 _ w325] -> w227
          event "Cancel": Value Change {
            n297 = event-data() -> ()  [unwired: 6 out]
            n298 = property on="Parameter" class="Str"() -> ("Value"=w231:string)  [unwired: 2 in, 2 out]
            n299 = property on="Interface" class="CmbBox"() -> ("Value"=w232:string)  [unwired: 2 in, 2 out]
            n300 = property on="Index Num" class="CmbBox"() -> ("Value"=w230:string)  [unwired: 2 in, 2 out]
            n301 = Build Array(w232, w231, w230) -> (w233:string[])
          }
          event "Interface": Value Change {
            n302 = event-data() -> ("NewVal"=w236:string)  [unwired: 6 out]
            n303 = case shown="\"RS232\"" w236 {
              tunnel: [_ _ _ TRUE ("可见") _ _] -> w235
              frame "GPIB", Default {
                w238 = FALSE
                w244 = FALSE
                w237 = FALSE
                n304 = property on="COM Port" class="CmbBox"("Visible"=w237) -> ()  [unwired: 2 in, 2 out]
                n305 = property on="Baud Rate" class="CmbBox"("Visible"=w237) -> ()  [unwired: 2 in, 2 out]
                n306 = property on="Parity" class="Ring (严格)"("Visible"=w237) -> ()  [unwired: 2 in, 2 out]
                n307 = property on="Data Bits" class="CmbBox"("Visible"=w237) -> ()  [unwired: 2 in, 2 out]
                n308 = property on="Stop Bits" class="CmbBox"("Visible"=w237) -> ()  [unwired: 2 in, 2 out]
                n309 = property on="IP" class="Str"("Visible"=w237) -> ()  [unwired: 2 in, 2 out]
                n310 = property on="Device Num" class="CmbBox"("Visible"=FALSE) -> ()  [unwired: 2 in, 2 out]
                n311 = property on="Index Num" class="CmbBox"("Visible"=TRUE) -> ()  [unwired: 2 in, 2 out]
                n312 = property on="GPIB Address" class="DigNum (严格)"("Visible"=TRUE) -> ()  [unwired: 2 in, 2 out]
                n313 = property on="VID" class="Str"("Visible"=w244) -> ()  [unwired: 2 in, 2 out]
                n314 = property on="PID" class="Str"("Visible"=w244) -> ()  [unwired: 2 in, 2 out]
                n315 = property on="SN" class="Str"("Visible"=w244) -> ()  [unwired: 2 in, 2 out]
                n316 = property on="IP" class="Str"("Visible"=w238) -> (error out=w241:errorcluster)  [unwired: 2 in, 1 out]
                n317 = property on="IP 2" class="Str"(error in=w241, "Visible"=w238) -> (error out=w240:errorcluster)  [unwired: 1 in, 1 out]
                n318 = property on="IP 3" class="Str"(error in=w240, "Visible"=w238) -> (error out=w239:errorcluster)  [unwired: 1 in, 1 out]
                n319 = property on="IP 4" class="Str"(error in=w239, "Visible"=w238) -> ()  [unwired: 1 in, 2 out]
              }
              frame "PCICard" {
                w247 = FALSE
                w254 = FALSE
                w246 = FALSE
                n320 = property on="VID" class="Str"("Visible"=w246) -> ()  [unwired: 2 in, 2 out]
                n321 = property on="PID" class="Str"("Visible"=w246) -> ()  [unwired: 2 in, 2 out]
                n322 = property on="SN" class="Str"("Visible"=w246) -> ()  [unwired: 2 in, 2 out]
                n323 = property on="Index Num" class="CmbBox"("Visible"=w246) -> ()  [unwired: 2 in, 2 out]
                n324 = property on="IP" class="Str"("Visible"=w246) -> ()  [unwired: 2 in, 2 out]
                n325 = property on="COM Port" class="CmbBox"("Visible"=w254) -> ()  [unwired: 2 in, 2 out]
                n326 = property on="Baud Rate" class="CmbBox"("Visible"=w254) -> ()  [unwired: 2 in, 2 out]
                n327 = property on="Parity" class="Ring (严格)"("Visible"=w254) -> ()  [unwired: 2 in, 2 out]
                n328 = property on="Data Bits" class="CmbBox"("Visible"=w254) -> ()  [unwired: 2 in, 2 out]
                n329 = property on="Stop Bits" class="CmbBox"("Visible"=w254) -> ()  [unwired: 2 in, 2 out]
                n330 = property on="IP" class="Str"("Visible"=w247) -> (error out=w250:errorcluster)  [unwired: 2 in, 1 out]
                n331 = property on="GPIB Address" class="DigNum (严格)"("Visible"=FALSE) -> ()  [unwired: 2 in, 2 out]
                n332 = property on="IP 2" class="Str"(error in=w250, "Visible"=w247) -> (error out=w249:errorcluster)  [unwired: 1 in, 1 out]
                n333 = property on="Device Num" class="CmbBox"("Visible"=TRUE) -> ()  [unwired: 2 in, 2 out]
                n334 = property on="Index Num" class="CmbBox"("Visible"=TRUE) -> ()  [unwired: 2 in, 2 out]
                n335 = property on="IP 3" class="Str"(error in=w249, "Visible"=w247) -> (error out=w248:errorcluster)  [unwired: 1 in, 1 out]
                n336 = property on="IP 4" class="Str"(error in=w248, "Visible"=w247) -> ()  [unwired: 1 in, 2 out]
              }
              frame "RS232" {
                w258 = FALSE
                w264 = FALSE
                w266 = TRUE
                n337 = property on="IP" class="Str"("Visible"=w258) -> (error out=w261:errorcluster)  [unwired: 2 in, 1 out]
                n338 = property on="Model Name" class="Str"() -> ("Value"=w257:string)  [unwired: 2 in, 2 out]
                n339 = property on="IP 2" class="Str"(error in=w261, "Visible"=w258) -> (error out=w260:errorcluster)  [unwired: 1 in, 1 out]
                n340 = property on="IP 3" class="Str"(error in=w260, "Visible"=w258) -> (error out=w259:errorcluster)  [unwired: 1 in, 1 out]
                n341 = Equal?(x=w257, y="Freescale") -> (x = y?=w255:bool)
                n342 = property on="IP 4" class="Str"(error in=w259, "Visible"=w258) -> ()  [unwired: 1 in, 2 out]
                n343 = property on="IP" class="Str"("Visible"=w255) -> ()  [unwired: 2 in, 2 out]
                n344 = property on="COM Port" class="CmbBox"("Visible"=w266) -> ()  [unwired: 2 in, 2 out]
                n345 = property on="Baud Rate" class="CmbBox"("Visible"=w266) -> ()  [unwired: 2 in, 2 out]
                n346 = property on="Parity" class="Ring (严格)"("Visible"=w266) -> ()  [unwired: 2 in, 2 out]
                n347 = property on="Data Bits" class="CmbBox"("Visible"=w266) -> ()  [unwired: 2 in, 2 out]
                n348 = property on="Stop Bits" class="CmbBox"("Visible"=w266) -> ()  [unwired: 2 in, 2 out]
                n349 = property on="Device Num" class="CmbBox"("Visible"=FALSE) -> ()  [unwired: 2 in, 2 out]
                n350 = property on="GPIB Address" class="DigNum (严格)"("Visible"=FALSE) -> ()  [unwired: 2 in, 2 out]
                n351 = property on="Index Num" class="CmbBox"("Visible"=TRUE) -> ()  [unwired: 2 in, 2 out]
                n352 = property on="VID" class="Str"("Visible"=w264) -> ()  [unwired: 2 in, 2 out]
                n353 = property on="PID" class="Str"("Visible"=w264) -> ()  [unwired: 2 in, 2 out]
                n354 = property on="SN" class="Str"("Visible"=w264) -> ()  [unwired: 2 in, 2 out]
              }
              frame "RS485" {
                w271 = FALSE
                w277 = FALSE
                w279 = TRUE
                n355 = property on="IP" class="Str"("Visible"=w271) -> (error out=w274:errorcluster)  [unwired: 2 in, 1 out]
                n356 = property on="Model Name" class="Str"() -> ("Value"=w270:string)  [unwired: 2 in, 2 out]
                n357 = property on="IP 2" class="Str"(error in=w274, "Visible"=w271) -> (error out=w273:errorcluster)  [unwired: 1 in, 1 out]
                n358 = property on="IP 3" class="Str"(error in=w273, "Visible"=w271) -> (error out=w272:errorcluster)  [unwired: 1 in, 1 out]
                n359 = Equal?(x=w270, y="Freescale") -> (x = y?=w268:bool)
                n360 = property on="IP 4" class="Str"(error in=w272, "Visible"=w271) -> ()  [unwired: 1 in, 2 out]
                n361 = property on="Stop Bits" class="CmbBox"("Visible"=w279) -> ()  [unwired: 2 in, 2 out]
                n362 = property on="COM Port" class="CmbBox"("Visible"=w279) -> ()  [unwired: 2 in, 2 out]
                n363 = property on="Baud Rate" class="CmbBox"("Visible"=w279) -> ()  [unwired: 2 in, 2 out]
                n364 = property on="Parity" class="Ring (严格)"("Visible"=w279) -> ()  [unwired: 2 in, 2 out]
                n365 = property on="Data Bits" class="CmbBox"("Visible"=w279) -> ()  [unwired: 2 in, 2 out]
                n366 = property on="IP" class="Str"("Visible"=w268) -> ()  [unwired: 2 in, 2 out]
                n367 = property on="Index Num" class="CmbBox"("Visible"=TRUE) -> ()  [unwired: 2 in, 2 out]
                n368 = property on="Device Num" class="CmbBox"("Visible"=FALSE) -> ()  [unwired: 2 in, 2 out]
                n369 = property on="GPIB Address" class="DigNum (严格)"("Visible"=FALSE) -> ()  [unwired: 2 in, 2 out]
                n370 = property on="VID" class="Str"("Visible"=w277) -> ()  [unwired: 2 in, 2 out]
                n371 = property on="PID" class="Str"("Visible"=w277) -> ()  [unwired: 2 in, 2 out]
                n372 = property on="SN" class="Str"("Visible"=w277) -> ()  [unwired: 2 in, 2 out]
              }
              frame "TCP" {
                w281 = TRUE
                w287 = FALSE
                w280 = FALSE
                n373 = property on="COM Port" class="CmbBox"("Visible"=w280) -> ()  [unwired: 2 in, 2 out]
                n374 = property on="Baud Rate" class="CmbBox"("Visible"=w280) -> ()  [unwired: 2 in, 2 out]
                n375 = property on="Parity" class="Ring (严格)"("Visible"=w280) -> ()  [unwired: 2 in, 2 out]
                n376 = property on="Data Bits" class="CmbBox"("Visible"=w280) -> ()  [unwired: 2 in, 2 out]
                n377 = property on="Stop Bits" class="CmbBox"("Visible"=w280) -> ()  [unwired: 2 in, 2 out]
                n378 = property on="IP" class="Str"("Visible"=w280) -> ()  [unwired: 2 in, 2 out]
                n379 = property on="Device Num" class="CmbBox"("Visible"=FALSE) -> ()  [unwired: 2 in, 2 out]
                n380 = property on="GPIB Address" class="DigNum (严格)"("Visible"=FALSE) -> ()  [unwired: 2 in, 2 out]
                n381 = property on="Index Num" class="CmbBox"("Visible"=TRUE) -> ()  [unwired: 2 in, 2 out]
                n382 = property on="IP" class="Str"("Visible"=w281) -> (error out=w284:errorcluster)  [unwired: 2 in, 1 out]
                n383 = property on="VID" class="Str"("Visible"=w287) -> ()  [unwired: 2 in, 2 out]
                n384 = property on="PID" class="Str"("Visible"=w287) -> ()  [unwired: 2 in, 2 out]
                n385 = property on="SN" class="Str"("Visible"=w287) -> ()  [unwired: 2 in, 2 out]
                n386 = property on="IP 2" class="Str"(error in=w284, "Visible"=w281) -> (error out=w283:errorcluster)  [unwired: 1 in, 1 out]
                n387 = property on="IP 3" class="Str"(error in=w283, "Visible"=w281) -> (error out=w282:errorcluster)  [unwired: 1 in, 1 out]
                n388 = property on="IP 4" class="Str"(error in=w282, "Visible"=w281) -> ()  [unwired: 1 in, 2 out]
              }
              frame "USB" {
                n389 = property on="Device Type" class="Str"() -> ("Value"=w298:string)  [unwired: 2 in, 2 out]
                n390 = property on="Model Name" class="Str"() -> ("Value"=w295:string)  [unwired: 2 in, 2 out]
                n391 = property on="Model Name" class="Str"() -> ("Value"=w291:string)  [unwired: 2 in, 2 out]
                n392 = Not Equal?(x=w298, y="CAN Card") -> (x != y?=w297:bool)
                n393 = Not Equal?(x=w295, y="DSO-2250 USB") -> (x != y?=w296:bool)
                n394 = Not Equal?(x=w295, y="DSO102") -> (x != y?=w293:bool)
                n395 = Equal?(x=w291, y="Freescale") -> (x = y?=w289:bool)
                n396 = Compound Arithmetic op=AND(w297, w296, w293) -> (w292:bool)
                n397 = property on="IP" class="Str"("Visible"=w289) -> ()  [unwired: 2 in, 2 out]
                n398 = case shown="真" w292 {
                  frame False {
                    w301 = FALSE
                    w305 = FALSE
                    n399 = property on="VID" class="Str"("Visible"=w305) -> ()  [unwired: 2 in, 2 out]
                    n400 = property on="PID" class="Str"("Visible"=w305) -> ()  [unwired: 2 in, 2 out]
                    n401 = property on="SN" class="Str"("Visible"=w305) -> ()  [unwired: 2 in, 2 out]
                    n402 = property on="Device Num" class="CmbBox"("Visible"=TRUE) -> ()  [unwired: 2 in, 2 out]
                    n403 = property on="COM Port" class="CmbBox"("Visible"=w301) -> ()  [unwired: 2 in, 2 out]
                    n404 = property on="Baud Rate" class="CmbBox"("Visible"=w301) -> ()  [unwired: 2 in, 2 out]
                    n405 = property on="Parity" class="Ring (严格)"("Visible"=w301) -> ()  [unwired: 2 in, 2 out]
                    n406 = property on="Data Bits" class="CmbBox"("Visible"=w301) -> ()  [unwired: 2 in, 2 out]
                    n407 = property on="Stop Bits" class="CmbBox"("Visible"=w301) -> ()  [unwired: 2 in, 2 out]
                    n408 = property on="GPIB Address" class="DigNum (严格)"("Visible"=FALSE) -> ()  [unwired: 2 in, 2 out]
                    n409 = property on="Index Num" class="CmbBox"("Visible"=TRUE) -> ()  [unwired: 2 in, 2 out]
                  }
                  frame True {
                    w306 = FALSE
                    w313 = FALSE
                    w314 = TRUE
                    n410 = property on="VID" class="Str"("Visible"=w314) -> ()  [unwired: 2 in, 2 out]
                    n411 = property on="PID" class="Str"("Visible"=w314) -> ()  [unwired: 2 in, 2 out]
                    n412 = property on="SN" class="Str"("Visible"=w314) -> ()  [unwired: 2 in, 2 out]
                    n413 = property on="Index Num" class="CmbBox"("Visible"=TRUE) -> ()  [unwired: 2 in, 2 out]
                    n414 = property on="IP" class="Str"("Visible"=w306) -> (error out=w309:errorcluster)  [unwired: 2 in, 1 out]
                    n415 = property on="COM Port" class="CmbBox"("Visible"=w313) -> ()  [unwired: 2 in, 2 out]
                    n416 = property on="Baud Rate" class="CmbBox"("Visible"=w313) -> ()  [unwired: 2 in, 2 out]
                    n417 = property on="Parity" class="Ring (严格)"("Visible"=w313) -> ()  [unwired: 2 in, 2 out]
                    n418 = property on="Data Bits" class="CmbBox"("Visible"=w313) -> ()  [unwired: 2 in, 2 out]
                    n419 = property on="Stop Bits" class="CmbBox"("Visible"=w313) -> ()  [unwired: 2 in, 2 out]
                    n420 = property on="IP 2" class="Str"(error in=w309, "Visible"=w306) -> (error out=w308:errorcluster)  [unwired: 1 in, 1 out]
                    n421 = property on="IP 3" class="Str"(error in=w308, "Visible"=w306) -> (error out=w307:errorcluster)  [unwired: 1 in, 1 out]
                    n422 = property on="GPIB Address" class="DigNum (严格)"("Visible"=FALSE) -> ()  [unwired: 2 in, 2 out]
                    n423 = property on="IP 4" class="Str"(error in=w307, "Visible"=w306) -> ()  [unwired: 1 in, 2 out]
                    n424 = property on="Device Num" class="CmbBox"("Visible"=FALSE) -> ()  [unwired: 2 in, 2 out]
                  }
                }
              }
            }
            n425 = property on="Address" class="CmbBox"("Visible"=w235) -> ()  [unwired: 2 in, 2 out]
          }
          event "OK": Value Change {
            n426 = event-data() -> ()  [unwired: 7 out]
            n427 = property on="Interface" class="CmbBox"() -> ("Value"=w328:string)  [unwired: 2 in, 2 out]
            n428 = case shown="\"RS232\"" w328 {
              tunnel: [w334 w344 w348 w361 w363 w364 w370] -> w326
              tunnel: "Baud Rate" -> [w333 w339 _ _ _ _ _]
              tunnel: "Data Bits" -> [w332 w340 _ _ _ _ _]
              tunnel: "Stop Bits" -> [w331 w341 _ _ _ _ _]
              tunnel: "Parity" -> [w330 w338 _ _ _ _ _]
              frame "RS232" {
                w335 = ","
                n429 = property on="COM Port" class="CmbBox"() -> ("Value"=w337:string)  [unwired: 2 in, 2 out]
                n430 = Number To Decimal String(number=w330) -> (decimal integer string=w336:string)  [unwired: 1 out]
                n431 = Concatenate Strings(w337, w335, w333, w335, w336, w335, w332, w335, w331) -> (w334:string)
              }
              frame "RS485" {
                w343 = ","
                n432 = property on="COM Port" class="CmbBox"() -> ("Value"=w346:string)  [unwired: 2 in, 2 out]
                n433 = Number To Decimal String(number=w338) -> (decimal integer string=w345:string)  [unwired: 1 out]
                n434 = Concatenate Strings(w346, w343, w339, w343, w345, w343, w340, w343, w341, w343, "Address") -> (w344:string)
              }
              frame "USB" {
                n435 = property on="Device Type" class="Str"() -> ("Value"=w347:string)  [unwired: 2 in, 2 out]
                n436 = case shown="\"False\", 默认" w347 {
                  tunnel: [w354 w360] -> w348
                  frame "False", Default {
                    w357 = ","
                    n437 = property on="Model Name" class="Str"() -> ("Value"=w351:string)  [unwired: 2 in, 2 out]
                    n438 = Equal?(x=w351, y="DSO-2250 USB") -> ()  [unwired: 1 out]
                    n439 = Equal?(x=w351, y="DSO102") -> (x = y?=w349:bool)
                    n440 = Concatenate Strings("VID", w357, "PID", w357, "SN") -> (w353:string)
                    n441 = property on="Device Num" class="CmbBox"() -> ("Value"=w352:string)  [unwired: 2 in, 2 out]
                    n442 = Select(t=w352, s=w349, f=w353) -> (s? t:f=w354:string)
                  }
                  frame "CAN Card", "DSO-2250 USB", "DSO102" {
                    n443 = property on="Device Num" class="CmbBox"() -> ("Value"=w360:string)  [unwired: 2 in, 2 out]
                  }
                }
              }
              frame "GPIB", Default {
                n444 = Number To Decimal String(number="GPIB Address") -> (decimal integer string=w361:string)  [unwired: 1 out]
              }
              frame "PCICard" {
                n445 = property on="Device Num" class="CmbBox"() -> ("Value"=w363:string)  [unwired: 2 in, 2 out]
              }
              frame "TCP" {
                w366 = "."
                n446 = property on="IP" class="Str"() -> ("Value"=w369:string)  [unwired: 2 in, 2 out]
                n447 = property on="IP 2" class="Str"() -> ("Value"=w368:string)  [unwired: 2 in, 2 out]
                n448 = property on="IP 3" class="Str"() -> ("Value"=w367:string)  [unwired: 2 in, 2 out]
                n449 = property on="IP 4" class="Str"() -> ("Value"=w365:string)  [unwired: 2 in, 2 out]
                n450 = Concatenate Strings(w369, w366, w368, w366, w367, w366, w365) -> (w364:string)
              }
              frame "CANCard" {
                n451 = property on="Device Num" class="CmbBox"() -> ("Value"=w370:string)  [unwired: 2 in, 2 out]
              }
            }
            n452 = property on="Interface" class="CmbBox"() -> ("Value"=w327:string)  [unwired: 2 in, 2 out]
            n453 = property on="Model Name" class="Str"() -> ("Value"=w324:string)  [unwired: 2 in, 2 out]
            n454 = Equal?(x=w324, y="Freescale") -> (x = y?=w322:bool)
            n455 = property on="Index Num" class="CmbBox"() -> ("Value"=w320:string)  [unwired: 2 in, 2 out]
            n456 = Select(t="IP", s=w322, f=w320) -> (s? t:f=w319:string)
            n457 = Build Array(w327, w326, w319) -> (w325:string[])
          }
        }
        "布尔 2" <- w228
        n458 = Wait (ms)(milliseconds to wait=u32 20) -> ()  [unwired: 1 out]
      }
    }
  }
  "Data out" <- w9
  n459 = while {
    shift-left: _ -> [w373]
    shift-right: [w374] -> _
    shift-left: _ -> [w377]
    shift-right: ["Bar"] -> _
    tunnel: w2 -> [w378]
    stop <- w371 stop-if-true
    n460 = Not(x=w377) -> (.not. x?=w376:bool)
    n461 = Wait (ms)(milliseconds to wait=u32 10) -> ()  [unwired: 1 out]
    n462 = And(x=w376, y="Bar") -> (x .and. y?=w372:bool)
    n463 = case shown="真" "Bar" {
      tunnel: w378 -> [_ w384]
      tunnel: [w380 w383] -> w374
      tunnel: w373 -> [w380 w381]
      tunnel: w372 -> [_ w382]
      frame False {
      }
      frame True {
        n464 = case shown="假" w382 {
          tunnel: w384 -> [w390 w406]
          tunnel: [w385 w396] -> w383
          tunnel: w381 -> [w385 _]
          frame False {
            n465 = Unbundle By Name(w385) -> ("x"=w393:i16, "y"=w392:i16)
            n466 = call "Get Cursor Position.vi"() -> ("cursor position"=w395:cluster{"x":i16, "y":i16})
            n467 = Unbundle By Name(w395) -> ("x"=w394:i16, "y"=w391:i16)
            n468 = Subtract(x=w394, y=w393) -> (x-y=w387:i16)
            n469 = Subtract(x=w391, y=w392) -> (x-y=w388:i16)
            n470 = Bundle By Name(cluster=cluster{"left":i16, "top":i16} {"left"=0, "top"=0} ("new position (0,0)"), "left"=w387, "top"=w388) -> (w386:cluster{"left":i16, "top":i16})
            n471 = call "Move Window.vi"("new position (0,0)"=w386, "window refnum (NaWR)"=w390) -> ()  [unwired: 2 in, 4 out]
          }
          frame True {
            n472 = call "Get Window Rectangle.vi"("window refnum (NaWR)"=w406) -> ("window rect"=w405:T2)  [unwired: 1 in, 5 out]
            n473 = call "Extract Window Origin.vi"("window rect"=w405) -> ("window origin"=w404:cluster{"left":i16, "top":i16})  [unwired: 1 out]
            n474 = Unbundle By Name(w404) -> ("left"=w401:i16, "top"=w400:i16)
            n475 = call "Get Cursor Position.vi"() -> ("cursor position"=w403:cluster{"x":i16, "y":i16})
            n476 = Unbundle By Name(w403) -> ("x"=w402:i16, "y"=w399:i16)
            n477 = Subtract(x=w402, y=w401) -> (x-y=w397:i16)
            n478 = Subtract(x=w399, y=w400) -> (x-y=w398:i16)
            n479 = Bundle By Name(cluster=w403, "x"=w397, "y"=w398) -> (w396:cluster{"x":i16, "y":i16})
          }
        }
      }
    }
    n480 = property on="布尔 2" class="Bool (严格)"() -> ("Value"=w371:bool)  [unwired: 2 in, 2 out]
  }
  n481 = property on="Address" class="CmbBox"("Visible"=FALSE ("可见")) -> ()  [unwired: 2 in, 2 out]
